vi "RT_Call Write.vi"(8 "error in":errorcluster, 10 "Data":u8, 11 "FPGA VI Reference In":T1) -> (0 "error out":errorcluster, 3 "FPGA VI Reference Out":T1)   [LabVIEW 2018]
uses:
  Data Def/RT_FPGA VI Reference.ctl
  <vilib>/Utility/error.llb/Error Cluster From Error Code.vi
  <vilib>/rvi/errors/niLvFpgaAdjustHostInterfaceError.vi
  <vilib>/rvi/interface/nirviReadWriteControl/nirviReadWriteControl.xnode
  <vilib>/rvi/interface/Simulation/niFpgaSimulationCallBeginRW.vi
  NiFpgaLv.dll
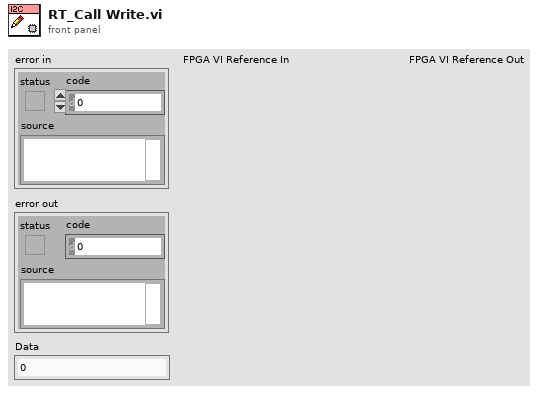
[diagram p1: front panel]
types:
  T1 = typedef "RT_FPGA VI Reference.ctl" = refnum<k20>
  T2 = enum16{"Idle", "Set Idle", "Config", "Read", "Write", "Arm", "Auto Run", "Auto Config", "Auto Write", "Auto Arm", "Auto Read", "Auto Check"}
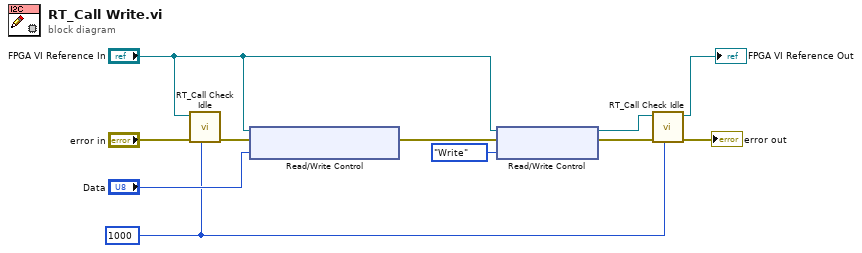
[diagram p0: block diagram]
diagram:
  w8 = 1000 ("Timeout?")
  n1 = call "RT_Call Check Idle.vi"("Timeout?"=w8, "error in"="error in", "FPGA VI Reference In"="FPGA VI Reference In") -> ("error out"=w7:errorcluster)  [unwired: 7 in, 1 out]
  n2 = xnode "Read/Write Control"("FPGA VI Reference In"="FPGA VI Reference In", "error in"=w7, "I2C Protocol Input Data"="Data") -> ("error out"=w6:errorcluster)  [unwired: 1 out]
  n3 = xnode "Read/Write Control"("FPGA VI Reference In"="FPGA VI Reference In", "error in"=w6, "I2C Loop State"=T2."Write") -> ("FPGA VI Reference Out"=w4:T1, "error out"=w5:errorcluster)
  n4 = call "RT_Call Check Idle.vi"("Timeout?"=w8, "error in"=w5, "FPGA VI Reference In"=w4) -> ("error out"=→"error out":errorcluster, "FPGA VI Reference Out"=→"FPGA VI Reference Out":T1)  [unwired: 7 in]
